vi "AcquireCameraImagesWithQueueAndWorkers.vi"() -> ()   [LabVIEW 2019]
doc: "The Parallel Processing (Optimized Performance) example shows how to process multiple images in parallel when using a ring acquisition. Images acquired from a camera are stored in a ring buffer and references to each image are pushed to a queue. Each worker loop removes a reference from the queue and processes the image.\n\nIn this example, image processing is simulated by a time delay that can be adjusted while the VI is running. When processing is complete, <B>IMAQdx Release Image</B> must be called in order to free space in the ring buffer."
uses:
  <vilib>/vision/driver/IMAQdx.llb/IMAQdx Acquisition Mode.ctl
  <vilib>/vision/Image Controls.llb/IMAQ Image.ctl
  <vilib>/vision/driver/IMAQdx.llb/IMAQdx Buffer Number Mode.ctl
  <vilib>/vision/driver/NI_Vision_Acquisition_Software.lvlib
  <resource>/objmgr/imaqdx.rc
panel:
  out "Lost Buffer Count":u32
  in  "Processing Delay (s)":dbl(slide)=0.1 scale=0.0..1.0
  out "Images Processed":u32
  out "Current Buffer Number":u32
  in  "Processing Delay (s)":dbl(slide)=0.2 scale=0.0..1.0
  out "Images Processed":u32
  out "Current Buffer Number":u32
  in  "Number of Images":i32=30
  out "Images in Queue":i32
  in  "Processing Delay (s)":dbl(slide)=0.4 scale=0.0..1.0
  out "Images Processed":u32
  out "Current Buffer Number":u32
  in  "Camera Name":refnum<k21> caption="IMAQdx Session"
  in  "Stop":bool
  # "Overview: Demonstrates how to process multiple extracted images in parallel when using a ring acquisition.\nRequirements: Vision Acquisition Software\nInstructions:\n1. Select the Camera Name\n2. Run the VI"
  # "Worker Loop 3"
  # "Worker Loop 2"
  # "Worker Loop 1"
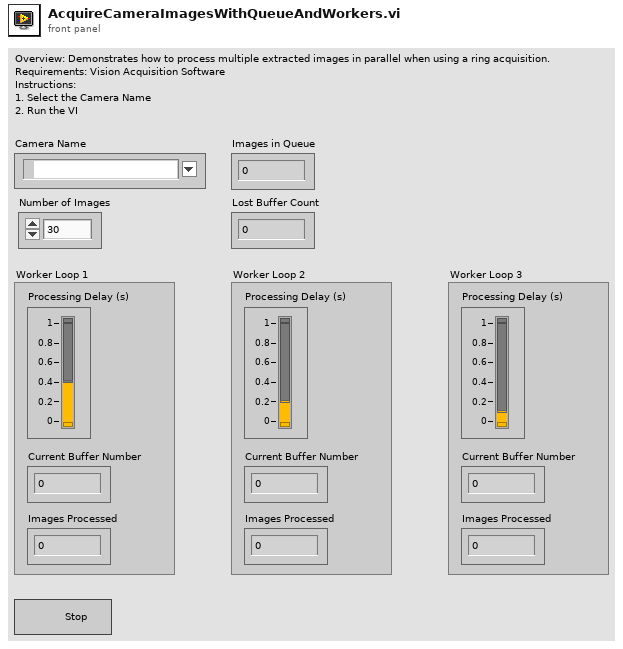
[diagram p1: front panel]
types:
  T1 = typedef "IMAQ Image.ctl" = refnum<image>
  T2 = typedef "NI_Vision_Acquisition_Software.lvlib/IMAQdx Acquisition Mode.ctl" = enum32{"One Shot", "Continuous"}
  T3 = typedef "IMAQdx.ctl" = refnum<k21>
  T4 = typedef "NI_Vision_Acquisition_Software.lvlib/IMAQdx Buffer Number Mode.ctl" = enum32{"Next", "Last", "Buffer Number", "Every", "Last New"}
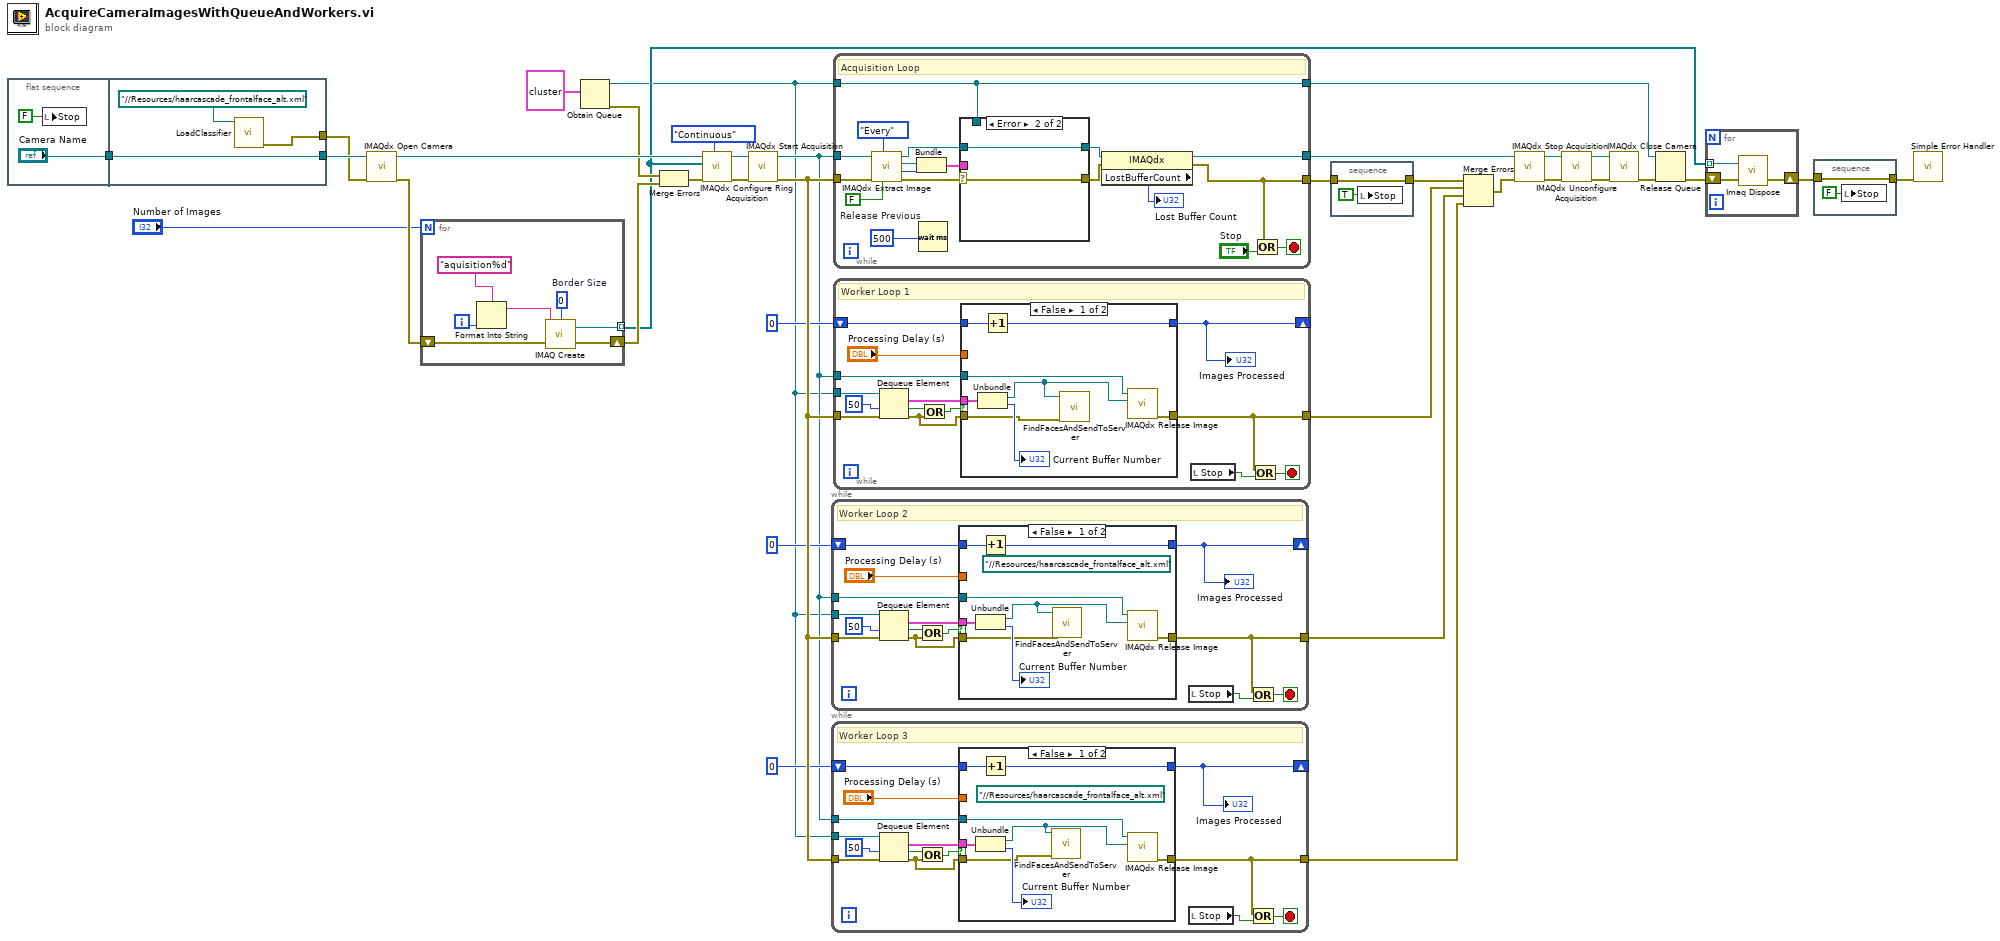
[diagram p0: block diagram]
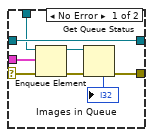
[diagram p5: hidden frame]
diagram:
  n1 = flat-sequence {
    tunnel: ["Camera Name"] -> w2
    tunnel: [w41] -> w32
    tunnel: w2 -> [w41]
    tunnel: [w39] -> w1
    frame #0 {
      n2 = local write "Stop"(FALSE ("Stop")) -> ()
    }
    frame #1 {
      n3 = call "LoadClassifier.vi"("faceCascadePath"=path "../../Resources/haarcascade_frontalface_alt.xml" ("Face Cascade Path")) -> ("error out"=w39:errorcluster)  [unwired: 10 in]
    }
  }
  n4 = call <vilib>:"IMAQdx Open Camera.vi"("error in"=w1, "Session In"=w32) -> ("error out"=w25:errorcluster, "Session Out"=w24:T3)  [unwired: 1 in, 7 out]
  n5 = for {
    N: "Number of Images" -> [_]
    tunnel: [w47] -> w14 mode=indexing
    shift-right: [w46] -> w20
    shift-left: w25 -> [w48]
    i -> [w45]
    w42 = 0  # Border Size
    n6 = Format Into String(format string="aquisition%d" ("Image Name"), w45) -> (resulting string=w44:string)  [unwired: 2 in, 1 out]
    n7 = call "IMAQ Create"("Border Size"=w42, "Image Name"=w44, "error in (no error)"=w48) -> ("New Image"=w47:T1, "error out"=w46:errorcluster)  [unwired: 1 in, 1 out]
  }
  n8 = Obtain Queue(element data type=cluster{"Image Out":T1, "Buffer Number Out":u32} {"Image Out"=refnum, "Buffer Number Out"=0}) -> (queue out=w7:refnum<queue>, error out=w19:errorcluster)  [unwired: 4 in, 1 out]
  n9 = Merge Errors(w19, w20) -> (w21:errorcluster)
  n10 = call <vilib>:"IMAQdx Configure Ring Acquisition.vi"("Mode"=IMAQdx_Acquisition_Mode."Continuous" ("Continuous?"), "error in"=w21, "Images"=w14, "Session In"=w24) -> ("error out"=w26:errorcluster, "Session Out"=w27:T3)  [unwired: 5 in, 1 out]
  n11 = call <vilib>:"IMAQdx Start Acquisition.vi"("error in"=w26, "Session In"=w27) -> ("error out"=w36:errorcluster, "Session Out"=w10:T3)  [unwired: 8 out]
  n12 = while {
    tunnel: [w55] -> w9
    tunnel: w7 -> [w59]
    tunnel: w10 -> [w58]
    shift-right: [w53] -> _
    shift-left: u32 0 -> [w57]
    tunnel: w36 -> [w52]
    stop <- w61 stop-if-true
    # "Worker Loop 2"
    n13 = Dequeue Element(queue=w59, timeout in ms (-1)=50 ("timeout in ms"), error in (no error)=w52) -> (element=w60:cluster{"Image Out":T1, "Buffer Number Out":u32}, timed out?=w49:bool, error out=w50:errorcluster)  [unwired: 1 out]
    n14 = Or(x=w49, y=w50) -> (x .or. y?=w51:bool)
    n15 = case shown="False" w51 {
      tunnel: w60 -> [w70 _]
      tunnel: [w69 w71] -> w55
      tunnel: "Processing Delay (s)" -> [_ _]
      tunnel: w58 -> [w68 _]
      tunnel: w57 -> [w67 w72]
      tunnel: [w66 w72] -> w53
      tunnel: w50 -> [w64 w71]
      frame False {
        (unwired) path "../../Resources/haarcascade_frontalface_alt.xml" ("Face Cascade Path")
        n16 = Unbundle(w70) -> ("Image Out"=w63:T1, "Buffer Number Out"=→"Current Buffer Number":u32)
        n17 = Increment(x=w67) -> (x+1=w66:u32)
        n18 = call "FindFacesAndSendToServer.vi"("error in"=w64, "Image In"=w63) -> ()  [unwired: 9 in, 1 out]
        n19 = call <vilib>:"IMAQdx Release Image.vi"("Image"=w63, "Session In"=w68) -> ("error out"=w69:errorcluster)  [unwired: 8 in, 1 out]
      }
      frame True {
        # "Empty queue or error.\nNothing to process."
      }
    }
    "Images Processed" <- w53
    n20 = local read "Stop"() -> (w56:bool)
    n21 = Or(x=w55, y=w56) -> (x .or. y?=w61:bool)
  }
  n22 = while {
    tunnel: [w79] -> w8
    tunnel: w7 -> [w83]
    tunnel: w10 -> [w82]
    shift-right: [w77] -> _
    shift-left: u32 0 -> [w81]
    tunnel: w36 -> [w76]
    stop <- w85 stop-if-true
    # "Worker Loop 3"
    n23 = Dequeue Element(queue=w83, timeout in ms (-1)=50 ("timeout in ms"), error in (no error)=w76) -> (element=w84:cluster{"Image Out":T1, "Buffer Number Out":u32}, timed out?=w75:bool, error out=w73:errorcluster)  [unwired: 1 out]
    n24 = Or(x=w75, y=w73) -> (x .or. y?=w74:bool)
    n25 = case shown="False" w74 {
      tunnel: w84 -> [w94 _]
      tunnel: [w93 w95] -> w79
      tunnel: "Processing Delay (s)" -> [_ _]
      tunnel: w82 -> [w92 _]
      tunnel: w81 -> [w91 w96]
      tunnel: [w90 w96] -> w77
      tunnel: w73 -> [w88 w95]
      frame False {
        (unwired) path "../../Resources/haarcascade_frontalface_alt.xml" ("Face Cascade Path")
        n26 = Unbundle(w94) -> ("Image Out"=w87:T1, "Buffer Number Out"=→"Current Buffer Number":u32)
        n27 = Increment(x=w91) -> (x+1=w90:u32)
        n28 = call "FindFacesAndSendToServer.vi"("error in"=w88, "Image In"=w87) -> ()  [unwired: 9 in, 1 out]
        n29 = call <vilib>:"IMAQdx Release Image.vi"("Image"=w87, "Session In"=w92) -> ("error out"=w93:errorcluster)  [unwired: 8 in, 1 out]
      }
      frame True {
        # "Empty queue or error.\nNothing to process."
      }
    }
    "Images Processed" <- w77
    n30 = local read "Stop"() -> (w80:bool)
    n31 = Or(x=w79, y=w80) -> (x .or. y?=w85:bool)
  }
  n32 = while {
    tunnel: w36 -> [w114]
    tunnel: w10 -> [w110]
    tunnel: w7 -> [w99]
    tunnel: [w109] -> w13
    tunnel: [w107] -> w6
    tunnel: [w99] -> w15
    stop <- w106 stop-if-true
    w111 = FALSE  # Release Previous
    # "Acquisition Loop"
    n33 = call <vilib>:"IMAQdx Extract Image.vi"("Release Previous (true)"=w111, "Buffer Number Mode (Next)"=IMAQdx_Buffer_Number_Mode."Every" ("Buffer Number Mode"), "error in"=w114, "Session In"=w110) -> ("error out"=w105:errorcluster, "Buffer Number Out"=w104:u32, "Image Out"=w103:T1, "Session Out"=w102:T3)  [unwired: 4 in]
    n34 = Bundle("Image Out"=w103, "Buffer Number Out"=w104) -> (w100:cluster{"Image Out":T1, "Buffer Number Out":u32})  [unwired: 1 in]
    n35 = Wait (ms)(milliseconds to wait=u32 500) -> ()  [unwired: 1 out]
    n36 = case shown="Error" w105 {
      selector: w105 -> [w118 w123]
      tunnel: [w119 w124] -> w101
      tunnel: w102 -> [w119 w124]
      tunnel: w100 -> [w117 _]
      tunnel: w99 -> [w116 _]
      tunnel: [w115 w123] -> w98
      frame No Error {
        n37 = Enqueue Element(queue=w116, element=w117, error in (no error)=w118) -> (queue out=w121:refnum<queue>, error out=w122:errorcluster)  [unwired: 1 in, 1 out]
        n38 = Get Queue Status(queue=w121, error in (no error)=w122) -> (error out=w115:errorcluster, # elements in queue=→"Images in Queue":i32)  [unwired: 1 in, 6 out]
      }
      frame Error {
      }
    }
    n39 = property class="IMAQdx"(reference=w101, error in=w98) -> (reference out=w109:T3, error out=w107:errorcluster, "LostBufferCount"=→"Lost Buffer Count":u32)
    n40 = Or(x=w107, y="Stop") -> (x .or. y?=w106:bool)
  }
  n41 = while {
    tunnel: [w130] -> w16
    tunnel: w7 -> [w134]
    tunnel: w10 -> [w133]
    shift-right: [w129] -> _
    shift-left: u32 0 -> [w132]
    tunnel: w36 -> [w128]
    stop <- w137 stop-if-true
    # "Worker Loop 1"
    n42 = Dequeue Element(queue=w134, timeout in ms (-1)=50 ("timeout in ms"), error in (no error)=w128) -> (element=w136:cluster{"Image Out":T1, "Buffer Number Out":u32}, timed out?=w126:bool, error out=w125:errorcluster)  [unwired: 1 out]
    n43 = Or(x=w126, y=w125) -> (x .or. y?=w127:bool)
    n44 = case shown="False" w127 {
      tunnel: w125 -> [w140 w148]
      tunnel: w136 -> [w146 _]
      tunnel: [w145 w148] -> w130
      tunnel: "Processing Delay (s)" -> [_ _]
      tunnel: w133 -> [w144 _]
      tunnel: w132 -> [w142 w147]
      tunnel: [w141 w147] -> w129
      frame False {
        n45 = Unbundle(w146) -> ("Image Out"=w139:T1, "Buffer Number Out"=→"Current Buffer Number":u32)
        n46 = Increment(x=w142) -> (x+1=w141:u32)
        n47 = call "FindFacesAndSendToServer.vi"("error in"=w140, "Image In"=w139) -> ()  [unwired: 9 in, 1 out]
        n48 = call <vilib>:"IMAQdx Release Image.vi"("Image"=w139, "Session In"=w144) -> ("error out"=w145:errorcluster)  [unwired: 8 in, 1 out]
      }
      frame True {
        # "Empty queue or error.\nNothing to process."
      }
    }
    "Images Processed" <- w129
    n49 = local read "Stop"() -> (w131:bool)
    n50 = Or(x=w130, y=w131) -> (x .or. y?=w137:bool)
  }
  n51 = stacked-sequence {
    tunnel: [w149] -> w5
    tunnel: w6 -> [w149]
    frame #0 {
      n52 = local write "Stop"(TRUE ("Stop")) -> ()
    }
  }
  n53 = Merge Errors(w5, w16, w9, w8) -> (w18:errorcluster)
  n54 = call <vilib>:"IMAQdx Stop Acquisition.vi"("error in"=w18, "Session In"=w13) -> ("error out"=w28:errorcluster, "Session Out"=w29:T3)  [unwired: 8 out]
  n55 = call <vilib>:"IMAQdx Unconfigure Acquisition.vi"("error in"=w28, "Session In"=w29) -> ("error out"=w31:errorcluster, "Session Out"=w30:T3)  [unwired: 8 out]
  n56 = call <vilib>:"IMAQdx Close Camera.vi"("error in"=w31, "Session In"=w30) -> ("error out"=w12:errorcluster)  [unwired: 9 out]
  n57 = Release Queue(queue=w15, error in (no error)=w12) -> (error out=w11:errorcluster)  [unwired: 1 in, 2 out]
  n58 = for {
    shift-right: [w152] -> w4
    shift-left: w11 -> [w153]
    tunnel: w14 -> [w151] mode=indexing
    n59 = call "Imaq Dispose"("Image"=w151, "error in (no error)"=w153) -> ("error out"=w152:errorcluster)  [unwired: 4 in]
  }
  n60 = stacked-sequence {
    tunnel: [w154] -> w3
    tunnel: w4 -> [w154]
    frame #0 {
      n61 = local write "Stop"(FALSE ("Stop")) -> ()
    }
  }
  n62 = call <vilib>:"Simple Error Handler.vi"("error in (no error)"=w3) -> ()  [unwired: 4 in, 5 out]
